vi "Sigma1.vi"(10 "Value":u32 format="0x%08x") -> (2 "Sigma 1":u32 format="0x%08x")   [LabVIEW 2018, in "Crypto.lvlib" / "SHA-256.lvclass"]
uses:
  SHA-256.lvclass
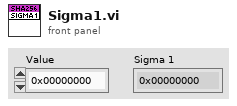
[diagram p1: front panel]
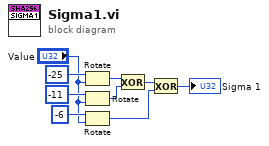
[diagram p0: block diagram]
diagram:
  n1 = Rotate(1:"Value", 2:i16 -25 ("y")) -> (0:w6:u32)
  n2 = Rotate(1:"Value", 2:i16 -11 ("y")) -> (0:w5:u32)
  n3 = Rotate(1:"Value", 2:i16 -6 ("y")) -> (0:w3:u32)
  n4 = Exclusive Or(1:w5, 2:w6) -> (0:w4:u32)
  n5 = Exclusive Or(1:w3, 2:w4) -> (0:→"Sigma 1":u32)
